vi "GetAppOutput.vi"(8 "error in (no error)":errorcluster, 11 "ModelValidation in":refnum<class "ModelValidationPlugin.lvclass">) -> (0 "error out":errorcluster, 3 "ModelValidation out":refnum<class "ModelValidationPlugin.lvclass">)   [LabVIEW 2014, in "AppPlugins.lvlib" / "ModelValidationPlugin.lvclass"]
uses:
  ModelValidationPlugin.lvclass
  TypeDef/Output.ctl
  AppPluginBaseClass/AppPluginsBase.lvclass/AppPluginsBase.ctl
  AppPluginBaseClass/Accessors/Read clEvtReportArray.vi
panel:
  out "Kalman gain":dbl[][](array[numeric])
  out "xk":dbl[][](array[numeric])
  out "Pk":dbl[][](array[numeric])
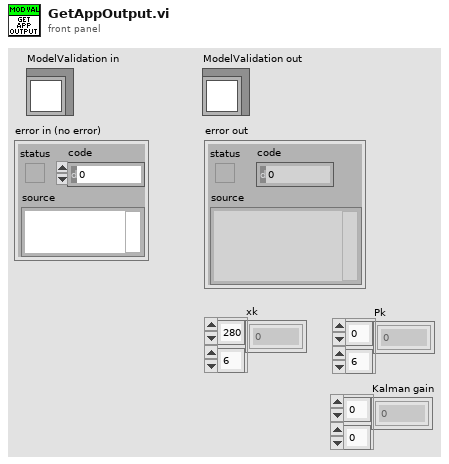
[diagram p1: front panel]
types:
  T1 = typedef "AppPlugins.lvlib/ModelValidationPlugin.lvclass/Output.ctl" = cluster{"xk":dbl[][], "Pk":dbl[][], "Kalman gain":dbl[][]}
  T2 = typedef "EventPlugins.lvlib/EventPluginBaseClass.lvclass/clEvtReportArray.ctl" = T3[]
  T3 = typedef "EventPlugins.lvlib/EventPluginBaseClass.lvclass/clEvtReport.ctl" = cluster{"Timestamp":dbl, "Synx":cdb[], "Freq":dbl, "ROCOF":dbl, "ID":i16}
  T4 = typedef "AppPlugins.lvlib/ModelValidationPlugin.lvclass/MatrixOutput.ctl" = cluster{"Fk":dbl[][], "zk":dbl[], "Hk":dbl[][], "Qk":dbl[][], "Rk":dbl[][]}
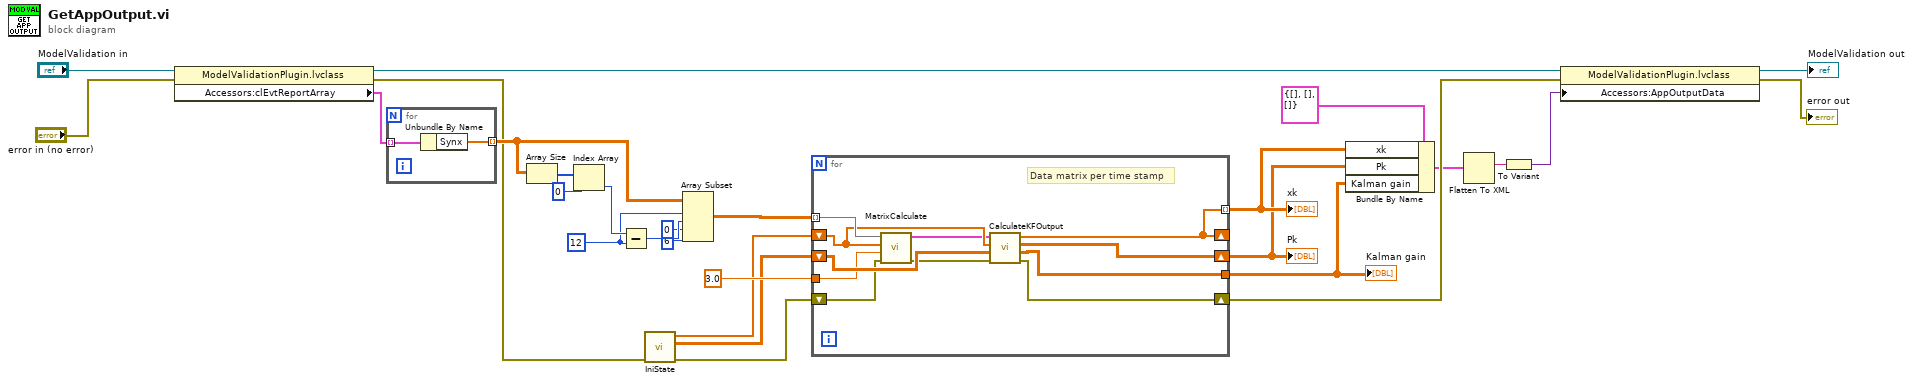
[diagram p0: block diagram]
diagram:
  w21 = 12 ("index")
  n1 = property class="ModelValidationPlugin.lvclass"(reference="ModelValidation in", error in="error in (no error)") -> (reference out=w7:refnum<class "ModelValidationPlugin.lvclass">, error out=w13:errorcluster, "Accessors:clEvtReportArray"=w28:T2)
  n2 = for {
    tunnel: [w30] -> w19 mode=indexing
    tunnel: w28 -> [w29] mode=indexing
    n3 = Unbundle By Name(w29) -> ("Synx"=w30:cdb[])
  }
  n4 = Array Size(array=w19) -> (size(s)=w24:i32[])
  n5 = Index Array(array=w24, index=0) -> (element=w22:i32)
  n6 = Subtract(x=w22, y=w21) -> (x-y=w18:i32)
  n7 = call "IniState.vi"("error in (no error)"=w13) -> ("error out"=w12:errorcluster, "Pk"=w14:dbl[][], "xk"=w15:dbl[])  [unwired: 8 in]
  n8 = Array Subset(array=w19, index (row)=w21, length (row)=w18, index (col)=0 ("index"), length (col)=6 ("length")) -> (w20:cdb[][])
  n9 = for {
    shift-right: [w36] -> w4
    shift-left: w12 -> [w37]
    tunnel: w20 -> [w41] mode=indexing
    shift-right: [w32] -> _
    shift-left: w15 -> [w35]
    shift-right: [w39] -> w9
    shift-left: w14 -> [w40]
    tunnel: 3.0 -> [w33]
    tunnel: [w32] -> w10 mode=indexing
    tunnel: [w31] -> w8
    # "Data matrix per time stamp"
    n10 = call "MatrixCalculate.vi"("error in (no error)"=w37, "I index"=w33, "xk"=w35, "Sync"=w41) -> ("error out"=w38:errorcluster, "output cluster"=w34:T4)  [unwired: 6 in]
    n11 = call "CalculateKFOutput.vi"("error in (no error)"=w38, "Pk"=w40, "xk"=w35, "MatrixCalculateOutput"=w34) -> ("error out"=w36:errorcluster, "Kalman gain"=w31:dbl[][], "Pk"=w39:dbl[][], "xk"=w32:dbl[])  [unwired: 4 in]
  }
  "Pk" <- w9
  "xk" <- w10
  "Kalman gain" <- w8
  n12 = Bundle By Name(cluster=T1 {"xk"=[], "Pk"=[], "Kalman gain"=[]} ("ModelValidationOutput"), "xk"=w10, "Pk"=w9, "Kalman gain"=w8) -> (w2:T1)
  n13 = Flatten To XML(anything=w2) -> (xml string=w3:string)
  n14 = To Variant(anything=w3) -> (Variant=w1:variant)
  n15 = property class="ModelValidationPlugin.lvclass"(reference=w7, error in=w4, "Accessors:AppOutputData"=w1) -> (reference out=→"ModelValidation out":refnum<class "ModelValidationPlugin.lvclass">, error out=→"error out":errorcluster)
